vi "Seq_Resume.vi"(8 "error in (no error)":errorcluster, 11 "Qbus in":refnum<class "Qbus.lvclass">) -> (0 "error out":errorcluster)   [LabVIEW 2016, in "SeqProcessor.lvlib"]
uses:
  SeqProcessor.lvlib
  <vilib>/addons/Qbus/Qbus.lvclass
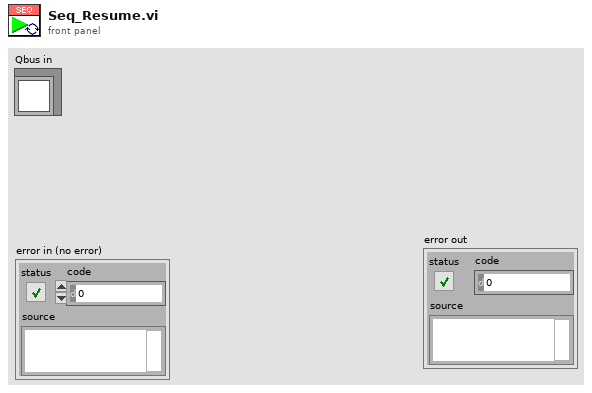
[diagram p1: front panel]
types:
  T1 = typedef "SeqProcessor.lvlib/StepIndex.ctl" = cluster{"Index1":u32, "Index2":u32}
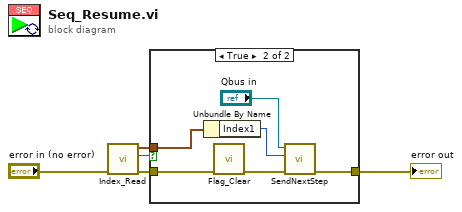
[diagram p0: block diagram]
diagram:
  n1 = call "Index_Read.vi"("error in (no error)"="error in (no error)") -> ("error out"=w1:errorcluster, "Found?"=w3:bool, "Index"=w2:T1)  [unwired: 8 in]
  n2 = case shown="True" w3 {
    tunnel: [w6 w11] -> w5
    tunnel: w2 -> [_ w8]
    tunnel: w1 -> [w6 w10]
    frame False {
    }
    frame True {
      n3 = Unbundle By Name(w8) -> ("Index1"=w7:u32)
      n4 = call "Flag_Clear.vi"("error in (no error)"=w10) -> ("error out"=w9:errorcluster)  [unwired: 10 in]
      n5 = call "SendNextStep.vi"("error in (no error)"=w9, "StepIndex"=w7, "Qbus in"="Qbus in") -> ("error out"=w11:errorcluster)  [unwired: 8 in]
    }
  }
  "error out" <- w5
